vi "BioFeedback23(v_0.4).vi"() -> ()   [LabVIEW 2016]
doc: "Use this template to build a producer/consumer design pattern. Use this template when you need to execute a process, such as data analysis, when a data source, such as a triggered acquisition, produces data at an uneven rate and you need to execute the process when the data becomes available."
uses:
  customSubVIs/8ChanWfmArray.ctl
  <vilib>/Utility/file.llb/Write Delimited Spreadsheet (string).vi
panel:
  out "RecordStartTime":timestamp
  out "startRecording":bool
  out "numChannels":dbl=20.0 caption="Lower Cut-Off"
  in  "Number of Channels":dbl=2.0 min=1.0 max=8.0 step=1.0
  out "DispQueueSize":dbl
  out "Display Values":dbl(graph)
  in  "Display Width for Data Stream":dbl(slide)=1.0 caption="Chart Width in Seconds" scale=0.1..10.0
  in  "infiniteTrial":bool=TRUE caption="Infinite Trial"
  out "MVC State":enum16{"Nothing", "Saved MVC", "NoSave MVC"}(ring)
  in  "MVC Delay (s)":dbl=3.0
  out "trial last time":timestamp
  out "mvc last time":timestamp
  in  "Display Width for MVC (s)":dbl(slide)=1.0 caption="Chart Width in Seconds" scale=0.1..10.0
  in  "Display Width for Current Trial":dbl(slide)=1.0 caption="Chart Width in Seconds" scale=0.1..10.0
  out "Current Trial (Filtered)":waveform(dbl)(graph)
  out "Current MVC (Filtered)":waveform(dbl)(graph)
  in  "enableSave":bool=TRUE caption="No Save      Save"
  in  "barOrGraph":bool=TRUE caption="Graph (under construction)       Bar"
  in  "Trial comment":string
  out "Collecting Data":bool
  in  "Display Min":dbl
  in  "Display Max":dbl=100.0
  in  "log filepath":path
  in  "Trial Duration (s)":dbl=3.0
  out "Trial Number":dbl
  in  "Session Name":string="Default"
  out "loopTime":dbl=30.0 caption="Upper Cut-Off"
  in  "trial display data":path
  out "Disp Data":cluster{"queue out":refnum<queue>, dbl, dbl}[](array[cluster])
  in  "Target Percentage":dbl=10.0
  out "Current Activation":dbl
  out "DisplayBarActivation":dbl(slide) caption="Percent Activation" max=1.0 scale=0.0..100.0
  in  "EMG Channel To Display":dbl=1.0
  out "MVC Data":cluster{"queue out":refnum<queue>, dbl, dbl}[](array[cluster])
  out "Trial Name":string="Test"
  in  "Data Directory":path=path "C:/Users/Tinggroup/Desktop/EMG Biofeedback System/LabviewFiles/Data"
  in  "MVC Number":dbl=3.0
  in  "MVC Duration (s)":dbl=3.0
  in  "Frames Per Second":dbl=30.0 caption="Upper Cut-Off"
  in  "EMG Input Device\nProduct Type":string="USB-6009"
  out "raw data":waveform(dbl)[](graph)
  out "dispSize":dbl=20.0 caption="Lower Cut-Off"
  out "mvcSize":dbl=300.0 caption="Upper Cut-Off"
  in  "MVC Window Size (s)":dbl=0.5
  in  "Display Window Size (s)":dbl=0.5
  in  "MVC Raw Path":path
  in  "trial raw data":path
  in  "trial filtered data":path
  in  "MVC Filtered Path":path
  in  "Sample rate (Hz)":dbl=1000.0 caption="Upper Cut-Off"
  out "fps":dbl=20.0 caption="Lower Cut-Off"
  out "rate":dbl=300.0 caption="Upper Cut-Off"
  in  "Set Parameters":bool
  out "lower":dbl=20.0 caption="Lower Cut-Off"
  out "upper":dbl=300.0 caption="Upper Cut-Off"
  in  "Lower Cut-Off":dbl=20.0
  in  "Upper Cut-Off":dbl=500.0
  in  "Mark":bool
  in  "End Trial":bool
  in  "Get MVC":bool
  in  "StartTrial":bool
  out "State":T1(ring)
  out "FilteredAndRectified":waveform(dbl)[](graph) caption="FilteredAndRectified Data By Channel"
  in  "stop":bool
  # "Behind The Scenes"
  # "Timing"
  # "Add trial comment\nBEFORE beginning trial"
  # "Off         On"
  # "Display Settings"
  # "Filtering"
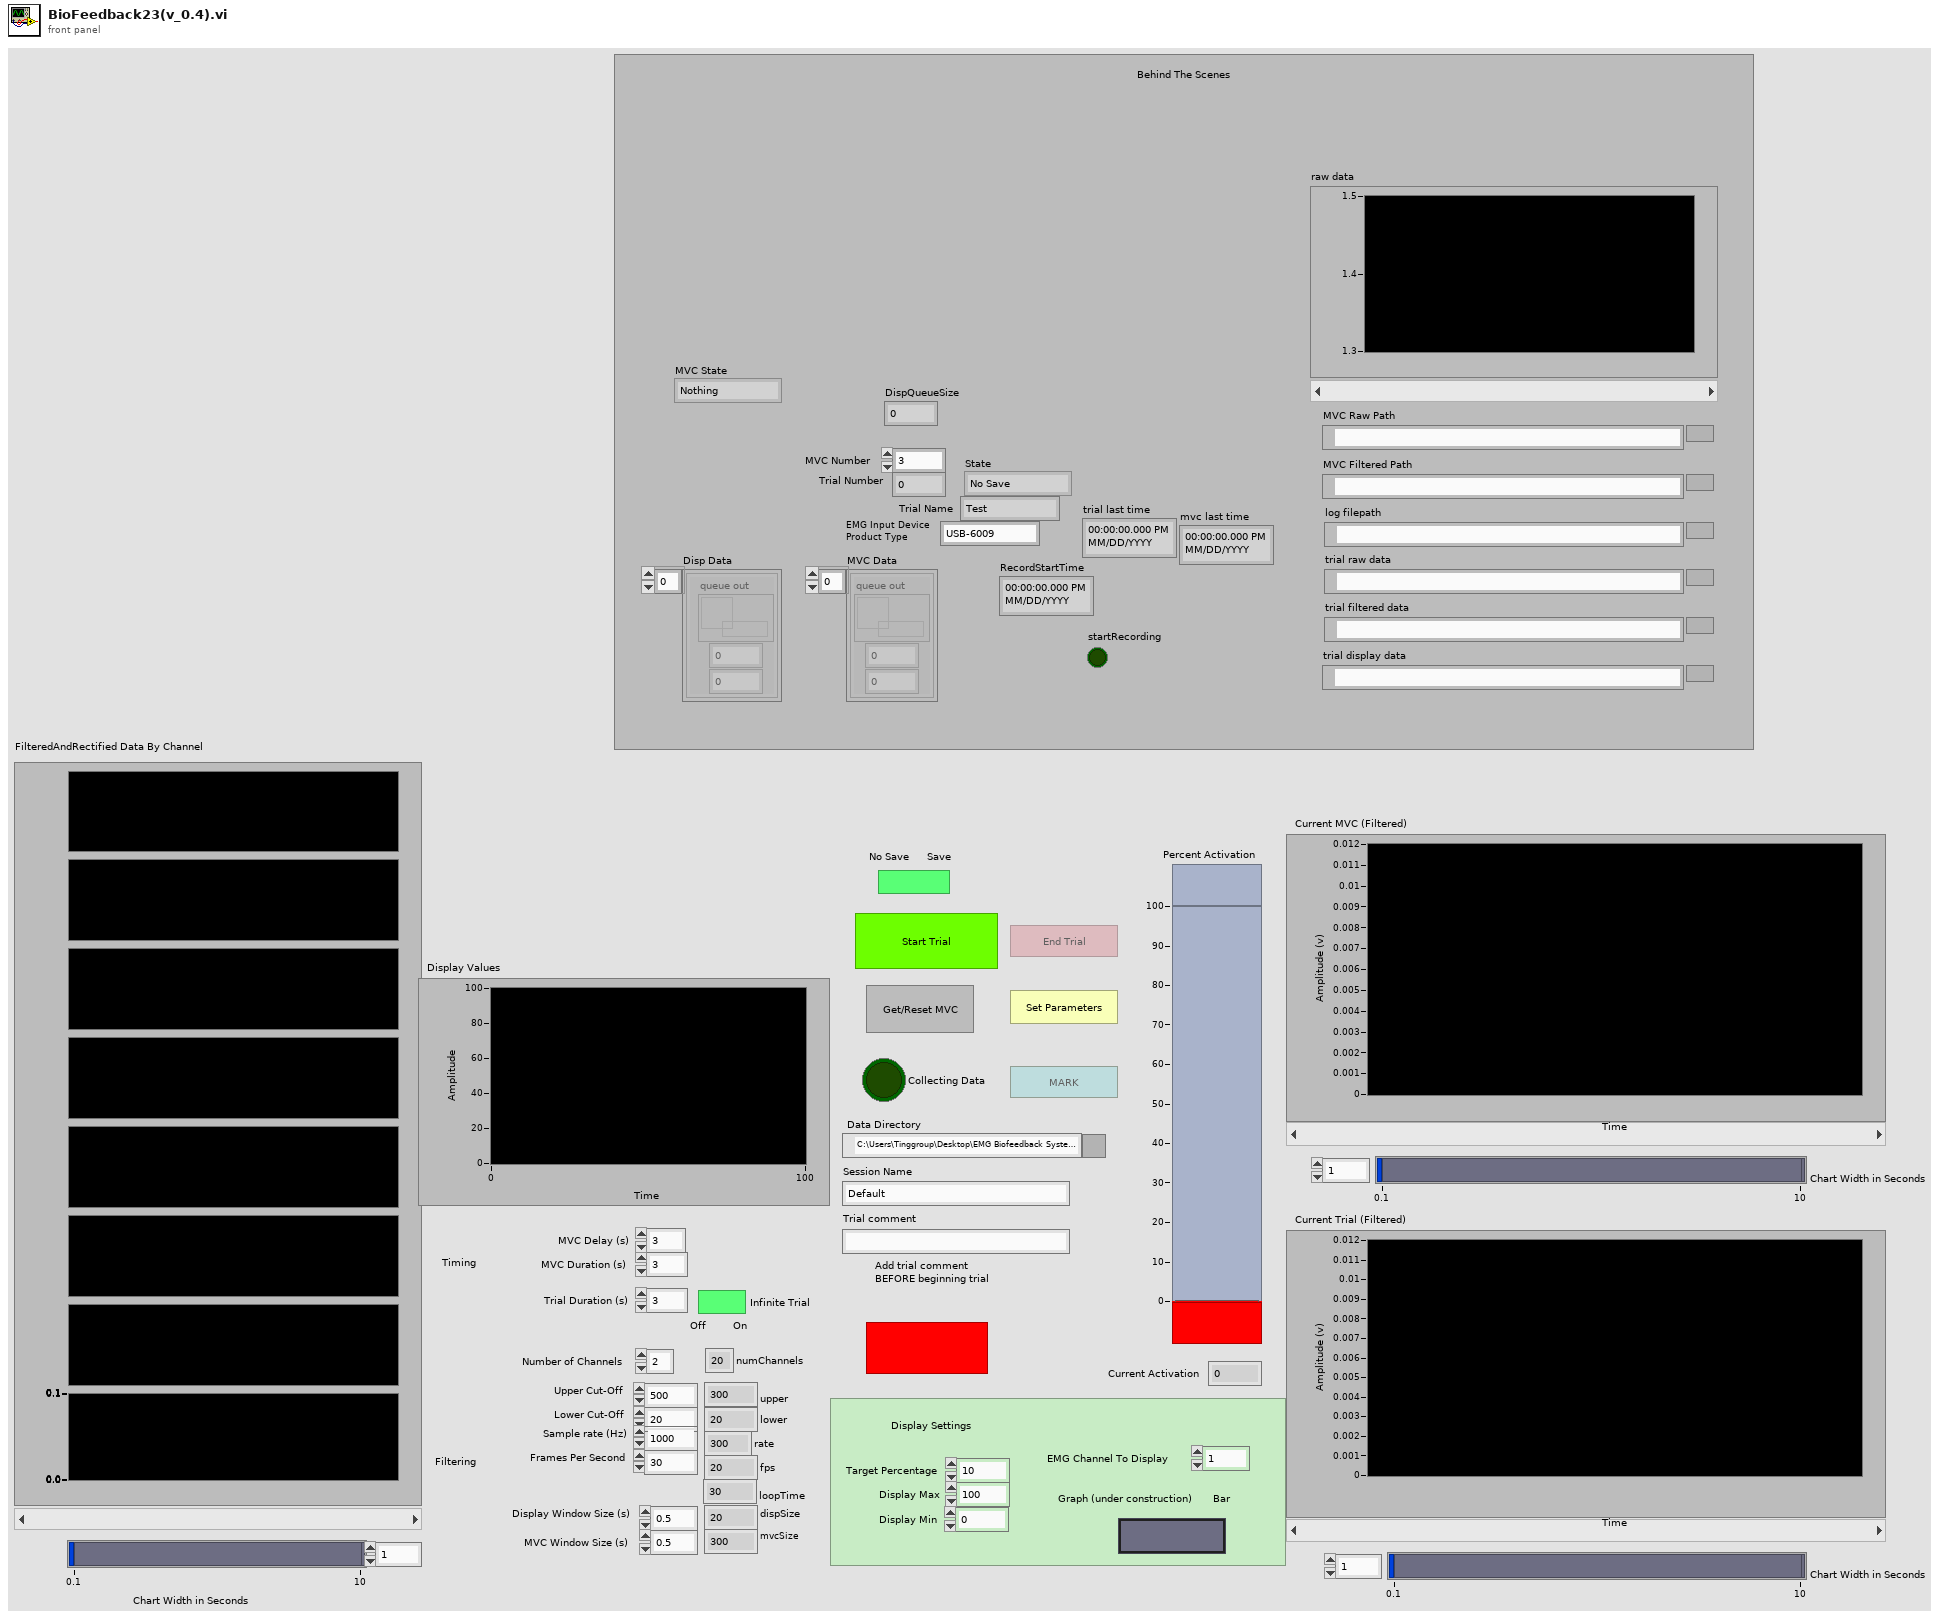
[diagram p1: front panel]
types:
  T1 = enum16{"No Save", "Acquiring Max", "Trial In Progress"}
  T2 = enum8{"Enabled", "Disabled", "Disabled and Grayed Out"}
  T3 = typedef "8ChanWfmArray.ctl" = waveform(dbl)[]
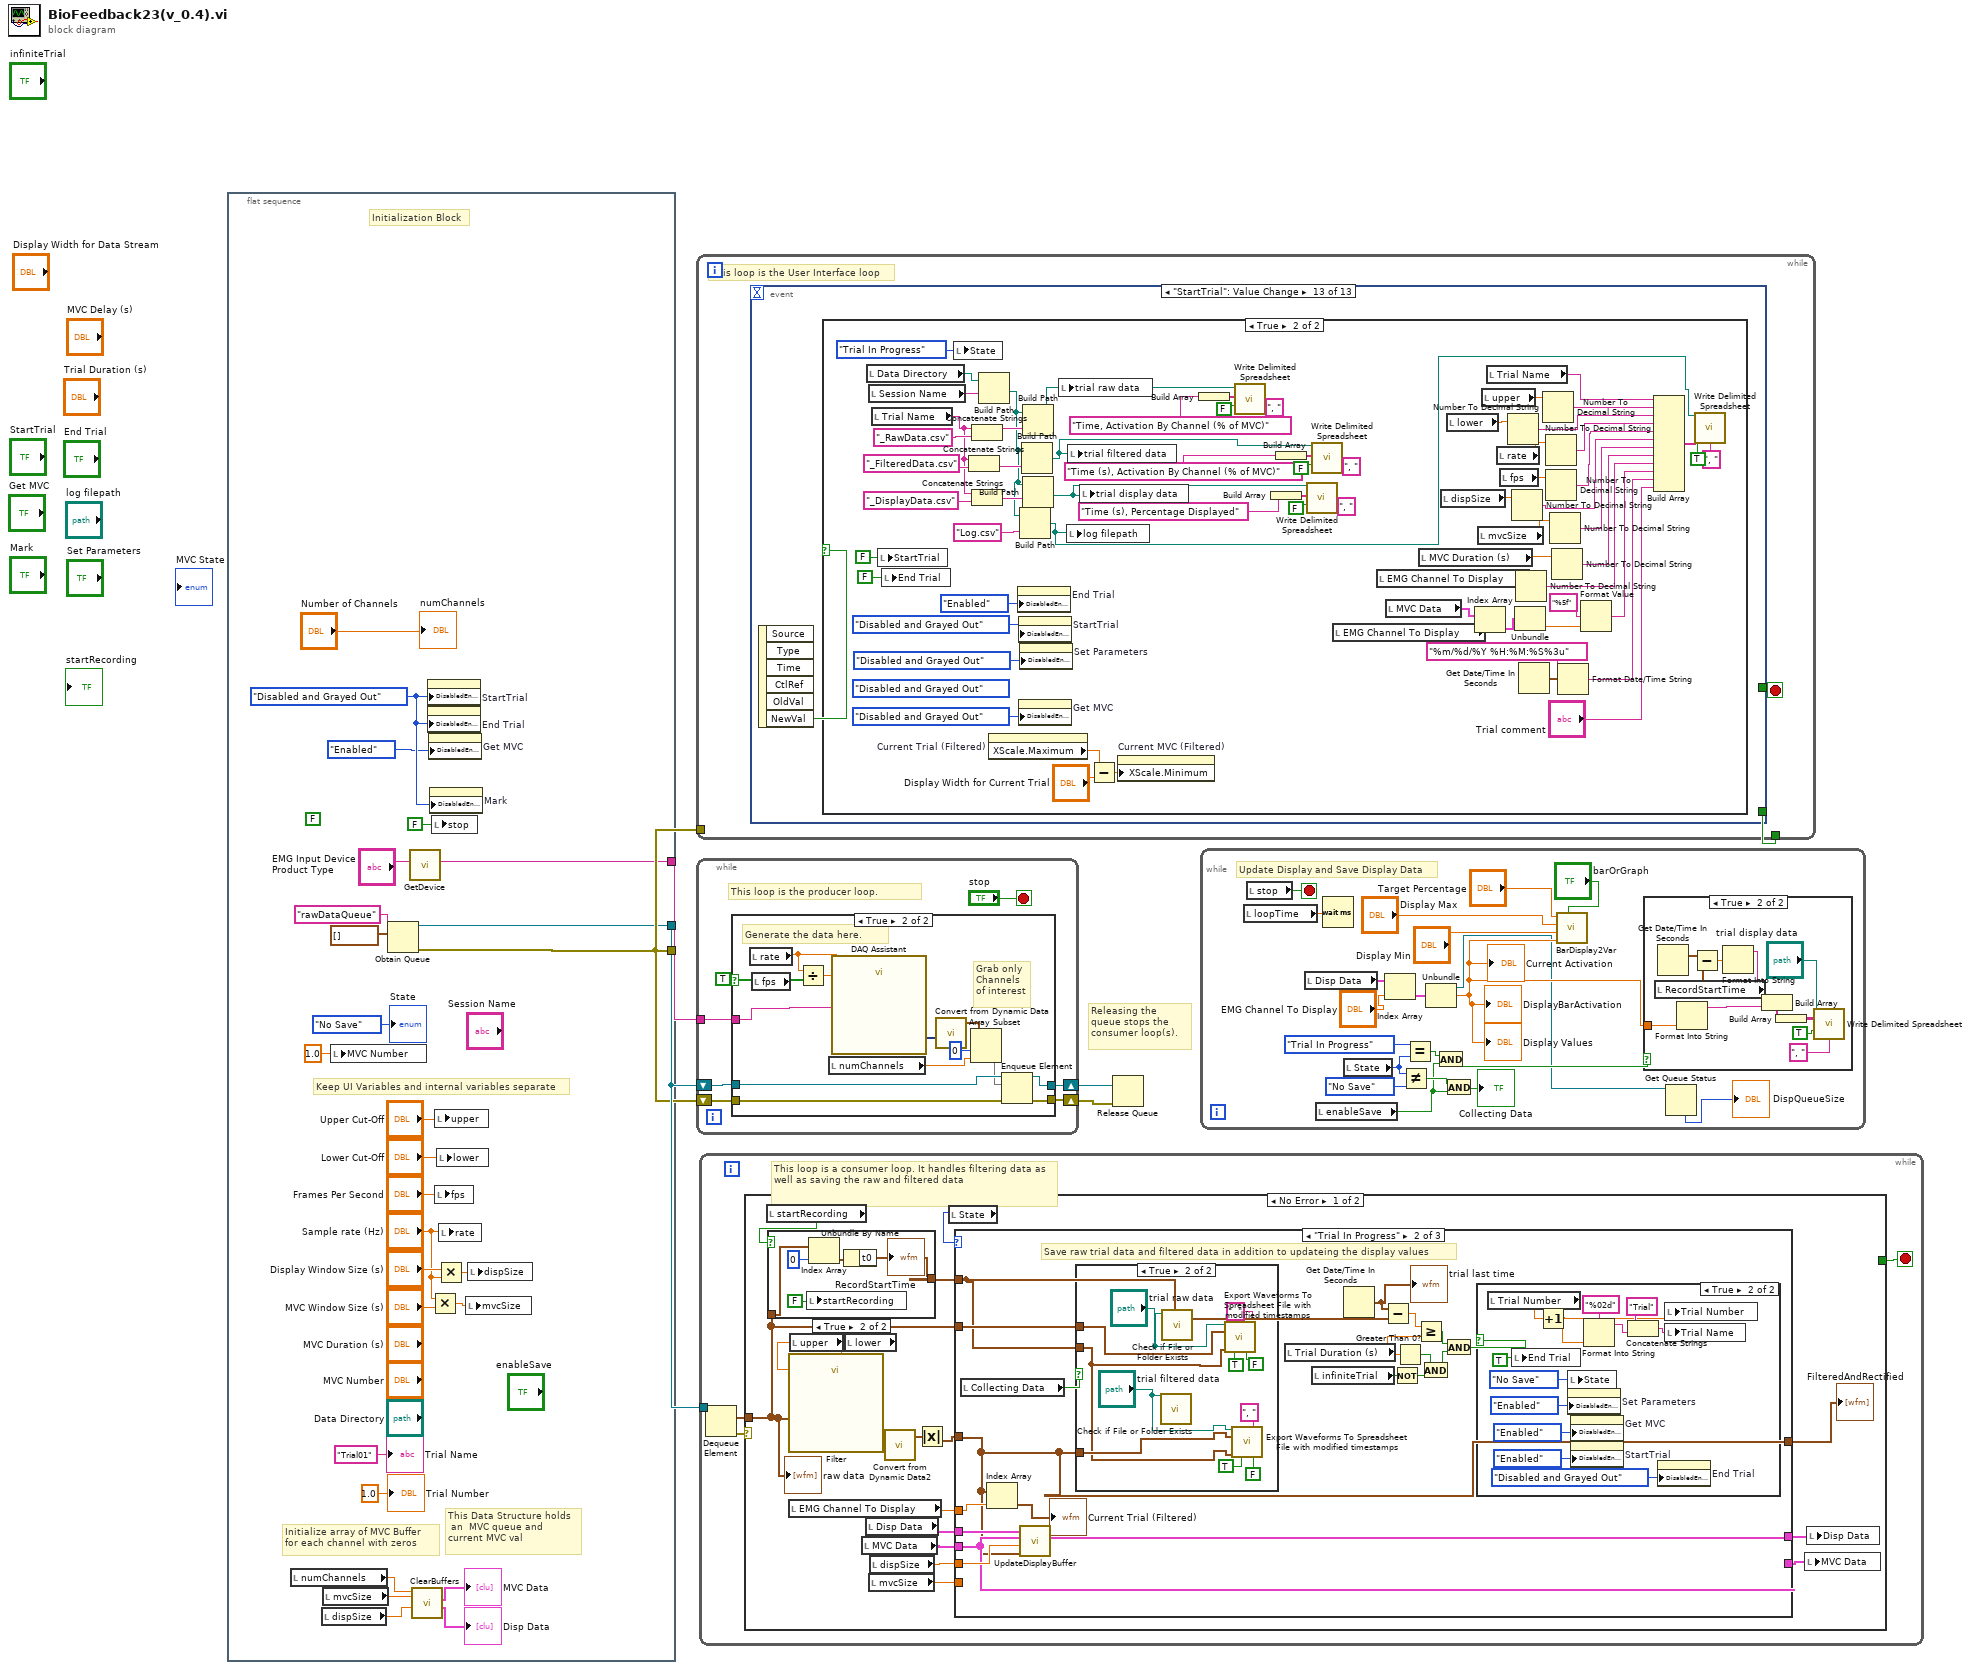
[diagram p0: block diagram]
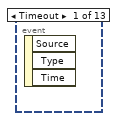
[diagram p3: hidden frame]
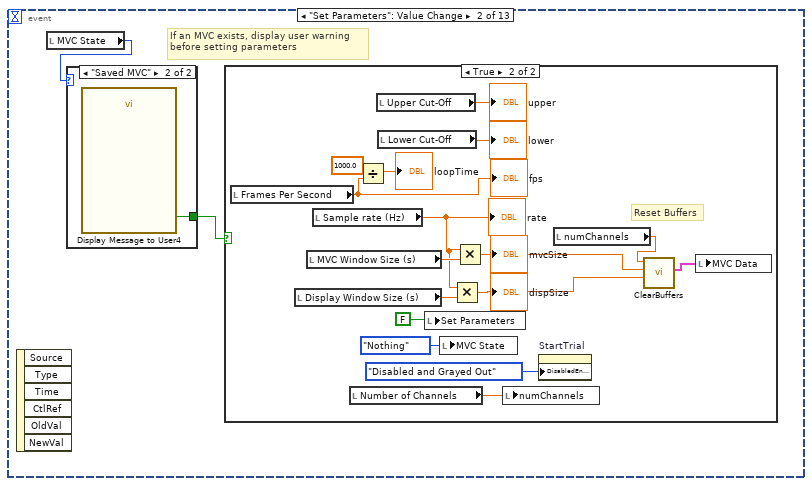
[diagram p4: hidden frame]
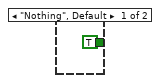
[diagram p6: hidden frame]
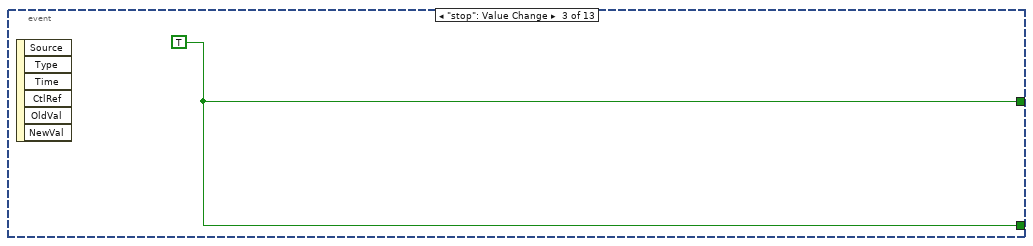
[diagram p7: hidden frame]
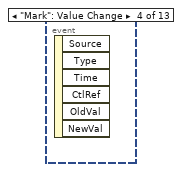
[diagram p8: hidden frame]
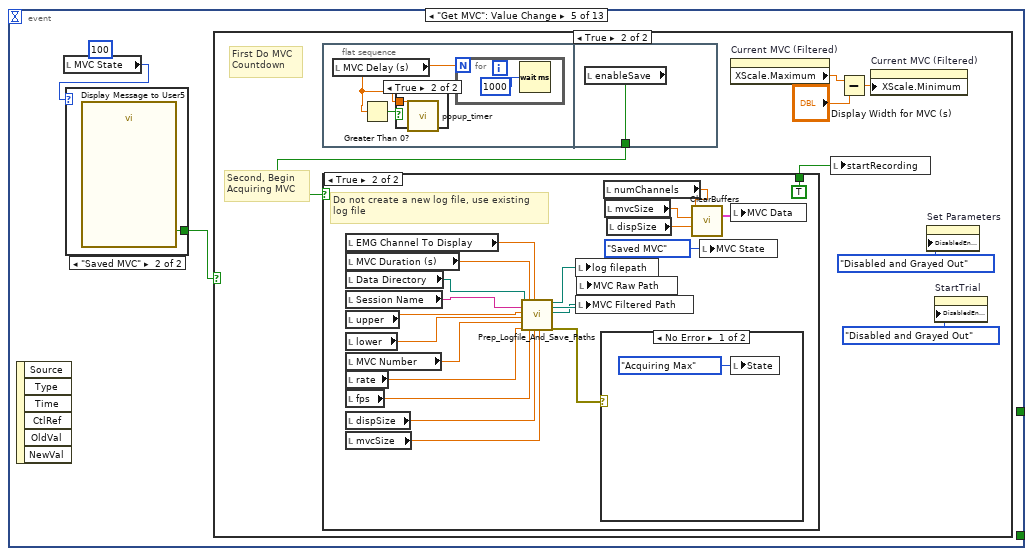
[diagram p9: hidden frame]
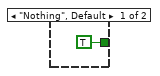
[diagram p10: hidden frame]
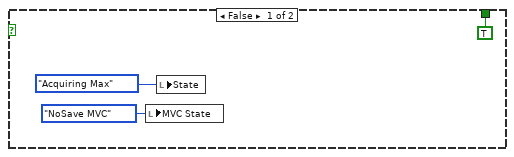
[diagram p13: hidden frame]
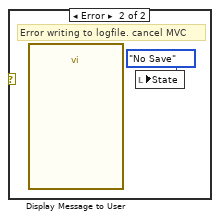
[diagram p14: hidden frame]
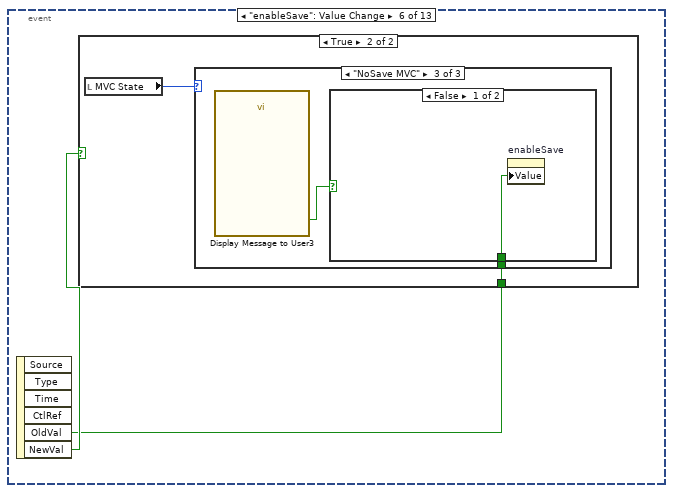
[diagram p15: hidden frame]
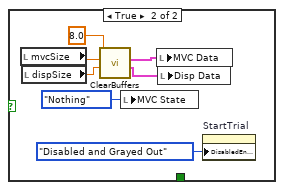
[diagram p19: hidden frame]
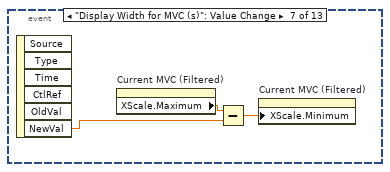
[diagram p20: hidden frame]
diagram:
  # "Releasing the\nqueue stops the consumer loop(s)."
  n1 = flat-sequence {
    tunnel: [w23] -> w2
    tunnel: [w22] -> w1
    tunnel: [w25] -> w3
    frame #0 {
      (unwired) FALSE ("Visible")
      w30 = T2."Disabled and Grayed Out" ("Disabled")
      # "Keep UI Variables and internal variables separate"
      # "This Data Structure holds\n an  MVC queue and \ncurrent MVC val"
      # "Initialize array of MVC Buffer \nfor each channel with zeros"
      # "Initialization Block"
      n2 = local read "numChannels"() -> (w6:dbl)
      n3 = local read "dispSize"() -> (w10:dbl)
      n4 = local read "mvcSize"() -> (w11:dbl)
      n5 = local write "MVC Number"(1.0 ("MVC Number")) -> ()
      n6 = Obtain Queue(name (unnamed)="rawDataQueue", element data type=T3 [] ("initialized array")) -> (queue out=w23:refnum<queue>, error out=w22:errorcluster)  [unwired: 3 in, 1 out]
      n7 = call "GetDevice.vi"("EMG Input Device\nProduct Type"="EMG Input Device\nProduct Type") -> ("DAQmx Device Name"=w25:tag)  [unwired: 10 in]
      n8 = call "ClearBuffers.vi"("disp size"=w10, "mvc size"=w11, "Num Channels"=w6) -> ("Disp Data"=→"Disp Data":cluster{"queue out":refnum<queue>, dbl, dbl}[], "MVC Data"=→"MVC Data":cluster{"queue out":refnum<queue>, dbl, dbl}[])  [unwired: 7 in]
      n9 = property on="StartTrial" class="Bool (strict)"("DisabledEnum"=w30) -> ()  [unwired: 2 in, 2 out]
      n10 = property on="End Trial" class="Bool (strict)"("DisabledEnum"=w30) -> ()  [unwired: 2 in, 2 out]
      n11 = property on="Get MVC" class="Bool"("DisabledEnum"=T2."Enabled" ("Disabled")) -> ()  [unwired: 2 in, 2 out]
      n12 = property on="Mark" class="Bool"("DisabledEnum"=w30) -> ()  [unwired: 2 in, 2 out]
      n13 = Multiply(x="Sample rate (Hz)", y="MVC Window Size (s)") -> (x*y=w17:dbl)
      n14 = local write "stop"(FALSE ("stop")) -> ()
      n15 = local write "upper"("Upper Cut-Off") -> ()
      n16 = local write "fps"("Frames Per Second") -> ()
      n17 = Multiply(x="Display Window Size (s)", y="Sample rate (Hz)") -> (x*y=w20:dbl)
      n18 = local write "lower"("Lower Cut-Off") -> ()
      n19 = local write "rate"("Sample rate (Hz)") -> ()
      n20 = local write "mvcSize"(w17) -> ()
      n21 = local write "dispSize"(w20) -> ()
      "Trial Name" <- "Trial01" ("Trial Name")
      "State" <- T1."No Save" ("State")
      "Trial Number" <- 1.0 ("Trial Number")
      "numChannels" <- "Number of Channels"
    }
  }
  n22 = while {
    tunnel: [w34] -> _
    tunnel: w1 -> [_]
    stop <- w33 stop-if-true
    # "This loop is the User Interface loop"
    n23 = event shown="[12] \"StartTrial\": Value Change" {
      selector: _ -> [_ _ _ _ _ _ _ _ _ _ _ _ _]
      dyn-events: _ -> [_ _ _ _ _ _ _ _ _ _ _ _ _]
      timeout: _ -> [_ _ _ _ _ _ _ _ _ _ _ _ _]
      tunnel: [_ _ w55 _ _ _ _ _ _ _ _ _ _] -> w33
      tunnel: [_ _ w55 _ _ _ _ _ _ _ _ _ _] -> w34
      event Timeout {
        n24 = event-data() -> ()  [unwired: 1 in, 3 out]
      }
      event "Set Parameters": Value Change {
        # "If an MVC exists, display user warning\nbefore setting parameters"
        n25 = event-data() -> ()  [unwired: 1 in, 6 out]
        n26 = local read "MVC State"() -> (w36:enum16{"Nothing", "Saved MVC", "NoSave MVC"})
        n27 = case shown="\"Saved MVC\"" w36 {
          tunnel: [TRUE ("Continue") w54] -> w35
          frame "Nothing", Default {
          }
          frame "Saved MVC" {
            n28 = call "Display Message to User4"() -> ("Continue"=w54:bool)  [unwired: 10 in, 1 out]
          }
        }
        n29 = case shown="True" w35 {
          frame False {
          }
          frame True {
            # "Reset Buffers"
            n30 = local read "Frames Per Second"() -> (w45:dbl)
            "fps" <- w45
            n31 = local read "Display Window Size (s)"() -> (w50:dbl)
            n32 = local read "MVC Window Size (s)"() -> (w51:dbl)
            n33 = local read "Sample rate (Hz)"() -> (w48:dbl)
            "rate" <- w48
            n34 = local read "Number of Channels"() -> (w37:dbl)
            n35 = Divide(x=1000.0, y=w45) -> (x/y=→"loopTime":dbl)
            n36 = local read "Upper Cut-Off"() -> (→"upper":dbl)
            n37 = local read "Lower Cut-Off"() -> (→"lower":dbl)
            n38 = local write "Set Parameters"(FALSE ("Set Parameters")) -> ()
            n39 = local write "MVC State"(enum16{"Nothing", "Saved MVC", "NoSave MVC"}."Nothing" ("MVC State")) -> ()
            n40 = Multiply(x=w48, y=w50) -> (x*y=w42:dbl)
            "dispSize" <- w42
            n41 = Multiply(x=w48, y=w51) -> (x*y=w43:dbl)
            "mvcSize" <- w43
            n42 = local write "numChannels"(w37) -> ()
            n43 = property on="StartTrial" class="Bool (strict)"("DisabledEnum"=T2."Disabled and Grayed Out" ("Disabled")) -> ()  [unwired: 2 in, 2 out]
            n44 = local read "numChannels"() -> (w38:dbl)
            n45 = call "ClearBuffers.vi"("disp size"=w42, "mvc size"=w43, "Num Channels"=w38) -> ("MVC Data"=w41:cluster{"queue out":refnum<queue>, dbl, dbl}[])  [unwired: 7 in, 1 out]
            n46 = local write "MVC Data"(w41) -> ()
          }
        }
      }
      event "stop": Value Change {
        w55 = TRUE
        n47 = event-data() -> ()  [unwired: 1 in, 6 out]
      }
      event "Mark": Value Change {
        n48 = event-data() -> ()  [unwired: 1 in, 6 out]
      }
      event "Get MVC": Value Change {
        (unwired) u32 100 ("milliseconds to wait")
        n49 = event-data() -> ()  [unwired: 1 in, 6 out]
        n50 = local read "MVC State"() -> (w57:enum16{"Nothing", "Saved MVC", "NoSave MVC"})
        n51 = case shown="\"Saved MVC\"" w57 {
          tunnel: [TRUE ("Continue") w59] -> w56
          frame "Nothing", Default {
          }
          frame "Saved MVC" {
            n52 = call "Display Message to User5"() -> ("Continue"=w59:bool)  [unwired: 10 in, 1 out]
          }
        }
        n53 = case shown="True" w56 {
          frame False {
          }
          frame True {
            # "Second, Begin \nAcquiring MVC"
            # "First Do MVC\nCountdown"
            n54 = flat-sequence {
              tunnel: [w71] -> w64
              frame #0 {
                n55 = local read "MVC Delay (s)"() -> (w67:dbl)
                n56 = Greater Than 0?(x=w67) -> (x > 0?=w68:bool)
                n57 = case shown="True" w68 {
                  tunnel: w67 -> [_ w69]
                  frame False {
                  }
                  frame True {
                    n58 = call "popup_timer.vi"("Seconds"=w69) -> ()  [unwired: 9 in, 1 out]
                  }
                }
                n59 = for {
                  N: w67 -> [_]
                  n60 = Wait (ms)(milliseconds to wait=u32 1000) -> ()  [unwired: 1 out]
                }
              }
              frame #1 {
                n61 = local read "enableSave"() -> (w71:bool)
              }
            }
            n62 = case shown="True" w64 {
              tunnel: [TRUE TRUE ("recordPressed")] -> w60
              frame False {
                n63 = local write "MVC State"(enum16{"Nothing", "Saved MVC", "NoSave MVC"}."NoSave MVC" ("MVC State")) -> ()
                n64 = local write "State"(T1."Acquiring Max" ("State")) -> ()
              }
              frame True {
                # "Do not create a new log file, use existing \nlog file"
                n65 = local read "EMG Channel To Display"() -> (w79:dbl)
                n66 = local read "MVC Duration (s)"() -> (w80:dbl)
                n67 = local read "Data Directory"() -> (w92:path)
                n68 = local read "Session Name"() -> (w91:string)
                n69 = local read "upper"() -> (w88:dbl)
                n70 = local read "lower"() -> (w87:dbl)
                n71 = local read "MVC Number"() -> (w86:dbl)
                n72 = local read "rate"() -> (w84:dbl)
                n73 = local read "fps"() -> (w83:dbl)
                n74 = local read "dispSize"() -> (w82:dbl)
                n75 = local read "mvcSize"() -> (w81:dbl)
                n76 = call "Prep_Logfile_And_Save_Paths.vi"("Data Directory"=w92, "Session Name"=w91, "upper"=w88, "lower"=w87, "MVC Number"=w86, "rate"=w84, "MVC Duration (s)"=w80, "fps"=w83, "EMG Channel To Display"=w79, "dispSize"=w82, "mvcSize"=w81) -> ("log filepath"=w90:path, "MVC Raw Path"=w89:path, "MVC Filtered Path"=w85:path, "error out"=w78:errorcluster)  [unwired: 4 in, 1 out]
                n77 = local write "log filepath"(w90) -> ()
                n78 = local write "MVC Filtered Path"(w85) -> ()
                n79 = local write "MVC Raw Path"(w89) -> ()
                n80 = case shown="No Error" w78 {
                  frame No Error {
                    n81 = local write "State"(T1."Acquiring Max" ("State")) -> ()
                  }
                  frame Error {
                    # "Error writing to logfile. cancel MVC"
                    n82 = call "Display Message to User"() -> ()  [unwired: 10 in, 2 out]
                    n83 = local write "State"(T1."No Save" ("State")) -> ()
                  }
                }
                n84 = local read "numChannels"() -> (w76:dbl)
                n85 = local read "mvcSize"() -> (w94:dbl)
                n86 = local read "dispSize"() -> (w93:dbl)
                n87 = call "ClearBuffers.vi"("disp size"=w93, "mvc size"=w94, "Num Channels"=w76) -> ("MVC Data"=w95:cluster{"queue out":refnum<queue>, dbl, dbl}[])  [unwired: 7 in, 1 out]
                n88 = local write "MVC State"(enum16{"Nothing", "Saved MVC", "NoSave MVC"}."Saved MVC" ("MVC State")) -> ()
                n89 = local write "MVC Data"(w95) -> ()
              }
            }
            n90 = property on="Current MVC (Filtered)" class="WFChart (strict)"() -> ("XScale.Maximum"=w61:dbl)  [unwired: 2 in, 2 out]
            n91 = local write "startRecording"(w60) -> ()
            n92 = Subtract(x=w61, y="Display Width for MVC (s)") -> (x-y=w63:dbl)
            n93 = property on="Current MVC (Filtered)" class="WFChart (strict)"("XScale.Minimum"=w63) -> ()  [unwired: 2 in, 2 out]
            n94 = property on="Set Parameters" class="Bool (strict)"("DisabledEnum"=T2."Disabled and Grayed Out" ("Disabled")) -> ()  [unwired: 2 in, 2 out]
            n95 = property on="StartTrial" class="Bool (strict)"("DisabledEnum"=T2."Disabled and Grayed Out" ("Disabled")) -> ()  [unwired: 2 in, 2 out]
          }
        }
      }
      event "enableSave": Value Change {
        n96 = event-data() -> ("OldVal"=w98:bool, "NewVal"=w99:bool)  [unwired: 1 in, 4 out]
        n97 = case shown="True" w99 {
          tunnel: w98 -> [_ w100]
          frame False {
          }
          frame True {
            n98 = local read "MVC State"() -> (w101:enum16{"Nothing", "Saved MVC", "NoSave MVC"})
            n99 = case shown="\"NoSave MVC\"" w101 {
              tunnel: w100 -> [_ _ w102]
              frame "Nothing", Default {
              }
              frame "Saved MVC" {
              }
              frame "NoSave MVC" {
                n100 = call "Display Message to User3"() -> ("Enable Saving"=w103:bool)  [unwired: 10 in, 1 out]
                n101 = case shown="False" w103 {
                  tunnel: w102 -> [w104 _]
                  frame False {
                    n102 = property on="enableSave" class="Bool (strict)"("Value"=w104) -> ()  [unwired: 2 in, 2 out]
                  }
                  frame True {
                    n103 = local read "mvcSize"() -> (w109:dbl)
                    n104 = local read "dispSize"() -> (w108:dbl)
                    n105 = call "ClearBuffers.vi"("disp size"=w108, "mvc size"=w109, "Num Channels"=8.0) -> ("Disp Data"=w111:cluster{"queue out":refnum<queue>, dbl, dbl}[], "MVC Data"=w110:cluster{"queue out":refnum<queue>, dbl, dbl}[])  [unwired: 7 in]
                    n106 = local write "MVC State"(enum16{"Nothing", "Saved MVC", "NoSave MVC"}."Nothing" ("MVC State")) -> ()
                    n107 = local write "MVC Data"(w110) -> ()
                    n108 = local write "Disp Data"(w111) -> ()
                    n109 = property on="StartTrial" class="Bool (strict)"("DisabledEnum"=T2."Disabled and Grayed Out" ("Disabled")) -> ()  [unwired: 2 in, 2 out]
                  }
                }
              }
            }
          }
        }
      }
      event "Display Width for MVC (s)": Value Change {
        n110 = event-data() -> ("NewVal"=w114:dbl)  [unwired: 1 in, 5 out]
        n111 = property on="Current MVC (Filtered)" class="WFChart (strict)"() -> ("XScale.Maximum"=w112:dbl)  [unwired: 2 in, 2 out]
        n112 = Subtract(x=w112, y=w114) -> (x-y=w113:dbl)
        n113 = property on="Current MVC (Filtered)" class="WFChart (strict)"("XScale.Minimum"=w113) -> ()  [unwired: 2 in, 2 out]
      }
      event "Display Width for Current Trial": Value Change {
        n114 = event-data() -> ("NewVal"=w117:dbl)  [unwired: 1 in, 5 out]
        n115 = property on="Current Trial (Filtered)" class="WFChart (strict)"() -> ("XScale.Maximum"=w115:dbl)  [unwired: 2 in, 2 out]
        n116 = Subtract(x=w115, y=w117) -> (x-y=w116:dbl)
        n117 = property on="Current Trial (Filtered)" class="WFChart (strict)"("XScale.Minimum"=w116) -> ()  [unwired: 2 in, 2 out]
      }
      event "Display Width for Data Stream": Value Change {
        n118 = event-data() -> ("NewVal"=w118:dbl)  [unwired: 1 in, 5 out]
        n119 = property on="raw data" class="WFChart (strict)"() -> ("XScale.Maximum"=w119:dbl)  [unwired: 2 in, 2 out]
        n120 = property on="FilteredAndRectified" class="WFChart (strict)"() -> ("XScale.Maximum"=w121:dbl)  [unwired: 2 in, 2 out]
        n121 = Subtract(x=w121, y=w118) -> (x-y=w120:dbl)
        n122 = Subtract(x=w119, y=w118) -> (x-y=w122:dbl)
        n123 = property on="raw data" class="WFChart (strict)"("XScale.Minimum"=w122) -> ()  [unwired: 2 in, 2 out]
        n124 = property on="FilteredAndRectified" class="WFChart (strict)"("XScale.Minimum"=w120) -> ()  [unwired: 2 in, 2 out]
      }
      event "infiniteTrial": Value Change {
        n125 = event-data() -> ("NewVal"=w123:bool)  [unwired: 1 in, 5 out]
        n126 = case shown="False" w123 {
          tunnel: [T2."Enabled" ("Disabled") T2."Disabled and Grayed Out" ("Disabled")] -> w124
          frame False {
          }
          frame True {
          }
        }
        n127 = property on="Trial Duration (s)" class="DigNum (strict)"("DisabledEnum"=w124) -> ()  [unwired: 2 in, 2 out]
      }
      event "Session Name": Value Change {
        # "Only Prompot if MVC already exists"
        # "Dialog Prompt User if they are sure that they want to change sessionname"
        n128 = event-data() -> ("OldVal"=w128:string)  [unwired: 1 in, 5 out]
        n129 = local read "MVC State"() -> (w127:enum16{"Nothing", "Saved MVC", "NoSave MVC"})
        n130 = case shown="\"Saved MVC\"" w127 {
          tunnel: w128 -> [_ w129]
          frame "Nothing", Default {
          }
          frame "Saved MVC" {
            n131 = call "Display Message to User2"() -> ("Change"=w130:bool)  [unwired: 10 in, 1 out]
            n132 = case shown="True" w130 {
              tunnel: w129 -> [w132 _]
              frame False {
                # "User cancels"
                n133 = Variant To Data(Variant=w132) -> (data=w131:string)  [unwired: 2 in, 1 out]
                n134 = local write "Session Name"(w131) -> ()
              }
              frame True {
                # "User Continues. Reset MVC"
                n135 = local read "numChannels"() -> (w133:dbl)
                n136 = local read "mvcSize"() -> (w138:dbl)
                n137 = local read "dispSize"() -> (w137:dbl)
                n138 = call "ClearBuffers.vi"("disp size"=w137, "mvc size"=w138, "Num Channels"=w133) -> ("Disp Data"=w135:cluster{"queue out":refnum<queue>, dbl, dbl}[], "MVC Data"=w136:cluster{"queue out":refnum<queue>, dbl, dbl}[])  [unwired: 7 in]
                n139 = local write "MVC State"(enum16{"Nothing", "Saved MVC", "NoSave MVC"}."Nothing" ("MVC State")) -> ()
                n140 = local write "MVC Data"(w136) -> ()
                n141 = local write "Disp Data"(w135) -> ()
                n142 = property on="StartTrial" class="Bool (strict)"("DisabledEnum"=T2."Disabled and Grayed Out" ("Disabled")) -> ()  [unwired: 2 in, 2 out]
              }
            }
          }
        }
      }
      event "End Trial": Value Change {
        n143 = event-data() -> ("NewVal"=w140:bool)  [unwired: 1 in, 5 out]
        n144 = case shown="True" w140 {
          frame False {
          }
          frame True {
            (unwired) T2."Enabled" ("Disabled")
            n145 = local read "Trial Number"() -> (w145:dbl)
            n146 = Increment(x=w145) -> (x+1=w141:dbl)
            n147 = local write "State"(T1."No Save" ("State")) -> ()
            n148 = Format Into String(format string="%02d", w141) -> (resulting string=w144:string)  [unwired: 2 in, 1 out]
            n149 = local write "Trial Number"(w141) -> ()
            n150 = Concatenate Strings("Trial" ("string"), w144) -> (w146:string)
            n151 = property on="End Trial" class="Bool (strict)"("DisabledEnum"=T2."Disabled and Grayed Out" ("Disabled")) -> ()  [unwired: 2 in, 2 out]
            n152 = property on="Get MVC" class="Bool"("DisabledEnum"=T2."Enabled" ("Disabled")) -> ()  [unwired: 2 in, 2 out]
            n153 = property on="Set Parameters" class="Bool (strict)"("DisabledEnum"=T2."Enabled" ("Disabled")) -> ()  [unwired: 2 in, 2 out]
            n154 = property on="StartTrial" class="Bool (strict)"("DisabledEnum"=T2."Enabled" ("Disabled")) -> ()  [unwired: 2 in, 2 out]
            n155 = local write "End Trial"(FALSE ("End Trial")) -> ()
            n156 = local write "Trial Name"(w146) -> ()
          }
        }
      }
      event "StartTrial": Value Change {
        n157 = event-data() -> ("NewVal"=w153:bool)  [unwired: 1 in, 5 out]
        n158 = case shown="True" w153 {
          frame False {
          }
          frame True {
            (unwired) T2."Disabled and Grayed Out" ("Disabled")
            n159 = local read "Data Directory"() -> (w213:path)
            n160 = local read "Session Name"() -> (w212:string)
            n161 = local read "Trial Name"() -> (w199:string)
            n162 = local write "StartTrial"(FALSE ("StartTrial")) -> ()
            n163 = local write "End Trial"(FALSE ("End Trial")) -> ()
            n164 = local write "State"(T1."Trial In Progress" ("State")) -> ()
            n165 = Concatenate Strings(w199, "_FilteredData.csv" ("string")) -> (w217:string)
            n166 = Concatenate Strings(w199, "_RawData.csv" ("string")) -> (w215:string)
            n167 = Concatenate Strings(w199, "_DisplayData.csv" ("string")) -> (w219:string)
            n168 = Build Path(base path=w213, name or relative path=w212) -> (appended path=w198:path)
            n169 = property on="Current Trial (Filtered)" class="WFChart (strict)"() -> ("XScale.Maximum"=w169:dbl)  [unwired: 2 in, 2 out]
            n170 = property on="End Trial" class="Bool (strict)"("DisabledEnum"=T2."Enabled" ("Disabled")) -> ()  [unwired: 2 in, 2 out]
            n171 = property on="StartTrial" class="Bool (strict)"("DisabledEnum"=T2."Disabled and Grayed Out" ("Disabled")) -> ()  [unwired: 2 in, 2 out]
            n172 = property on="Get MVC" class="Bool"("DisabledEnum"=T2."Disabled and Grayed Out" ("Disabled")) -> ()  [unwired: 2 in, 2 out]
            n173 = Build Path(base path=w198, name or relative path="Log.csv" ("string")) -> (appended path=w182:path)
            n174 = property on="Set Parameters" class="Bool (strict)"("DisabledEnum"=T2."Disabled and Grayed Out" ("Disabled")) -> ()  [unwired: 2 in, 2 out]
            n175 = Build Path(base path=w198, name or relative path=w217) -> (appended path=w160:path)
            n176 = Build Path(base path=w198, name or relative path=w215) -> (appended path=w164:path)
            n177 = Build Path(base path=w198, name or relative path=w219) -> (appended path=w155:path)
            n178 = local write "trial raw data"(w164) -> ()
            n179 = local write "log filepath"(w182) -> ()
            n180 = local write "trial filtered data"(w160) -> ()
            n181 = local write "trial display data"(w155) -> ()
            n182 = Subtract(x=w169, y="Display Width for Current Trial") -> (x-y=w171:dbl)
            n183 = property on="Current MVC (Filtered)" class="WFChart (strict)"("XScale.Minimum"=w171) -> ()  [unwired: 2 in, 2 out]
            n184 = Build Array("Time, Activation By Channel (% of MVC)" ("time format string (%c)")) -> (w166:string[])
            n185 = call-poly <vilib>:"Write Delimited Spreadsheet.vi"("file path (dialog if empty)"=w164, "1D data"=w166, "append to file? (new file:F)"=FALSE, "delimiter (\\t)"=", " ("delimiter (\\t)")) -> ()  [unwired: 10 in, 2 out]
            n186 = Build Array("Time (s), Percentage Displayed" ("time format string (%c)")) -> (w156:string[])
            n187 = Build Array("Time (s), Activation By Channel (% of MVC)" ("time format string (%c)")) -> (w161:string[])
            n188 = call-poly <vilib>:"Write Delimited Spreadsheet.vi"("file path (dialog if empty)"=w155, "1D data"=w156, "append to file? (new file:F)"=FALSE, "delimiter (\\t)"=", " ("delimiter (\\t)")) -> ()  [unwired: 10 in, 2 out]
            n189 = call-poly <vilib>:"Write Delimited Spreadsheet.vi"("file path (dialog if empty)"=w160, "1D data"=w161, "append to file? (new file:F)"=FALSE, "delimiter (\\t)"=", " ("delimiter (\\t)")) -> ()  [unwired: 10 in, 2 out]
            n190 = local read "EMG Channel To Display"() -> (w178:dbl)
            n191 = local read "EMG Channel To Display"() -> (w208:dbl)
            n192 = local read "MVC Data"() -> (w179:cluster{"queue out":refnum<queue>, dbl, dbl}[])
            n193 = local read "MVC Duration (s)"() -> (w207:dbl)
            n194 = local read "dispSize"() -> (w205:dbl)
            n195 = local read "lower"() -> (w202:dbl)
            n196 = Index Array(array=w179, index=w178) -> (element=w177:cluster{"queue out":refnum<queue>, dbl, dbl})
            n197 = local read "mvcSize"() -> (w206:dbl)
            n198 = local read "upper"() -> (w201:dbl)
            n199 = local read "Trial Name"() -> (w195:string)
            n200 = local read "rate"() -> (w203:dbl)
            n201 = local read "fps"() -> (w204:dbl)
            n202 = Number To Decimal String(number=w202) -> (decimal integer string=w191:string)  [unwired: 1 in]
            n203 = Number To Decimal String(number=w205) -> (decimal integer string=w189:string)  [unwired: 1 in]
            n204 = Unbundle(w177) -> (w173:dbl)  [unwired: 2 out]
            n205 = Number To Decimal String(number=w208) -> (decimal integer string=w186:string)  [unwired: 1 in]
            n206 = Get Date/Time In Seconds() -> (seconds since 1Jan1904=w181:timestamp)
            n207 = Number To Decimal String(number=w201) -> (decimal integer string=w192:string)  [unwired: 1 in]
            n208 = Number To Decimal String(number=w203) -> (decimal integer string=w190:string)  [unwired: 1 in]
            n209 = Number To Decimal String(number=w204) -> (decimal integer string=w185:string)  [unwired: 1 in]
            n210 = Number To Decimal String(number=w206) -> (decimal integer string=w188:string)  [unwired: 1 in]
            n211 = Number To Decimal String(number=w207) -> (decimal integer string=w187:string)  [unwired: 1 in]
            n212 = Format Date/Time String(time format string (%c)="%m/%d/%Y %H:%M:%S%3u", seconds (now)=w181) -> (date/time string=w176:string)  [unwired: 1 in]
            n213 = Format Value(format string="%5f", value (0)=w173) -> (output string=w172:string)  [unwired: 1 in]
            n214 = Build Array(w195, w192, w191, w190, w185, w189, w188, w187, w186, w172, w176, "Trial comment") -> (w184:string[])
            n215 = call-poly <vilib>:"Write Delimited Spreadsheet.vi"("file path (dialog if empty)"=w182, "1D data"=w184, "append to file? (new file:F)"=TRUE, "delimiter (\\t)"=", " ("delimiter (\\t)")) -> ()  [unwired: 10 in, 2 out]
          }
        }
      }
    }
  }
  n216 = while {
    shift-right: [w224] -> w4
    shift-left: w1 -> [w225]
    shift-right: [w221] -> w5
    shift-left: w2 -> [w226]
    tunnel: w3 -> [w222]
    stop <- "stop" stop-if-true
    # "This loop is the producer loop."
    n217 = case shown="True" TRUE ("Case Constant\n(See Context Help)") {
      tunnel: w226 -> [w228 w237]
      tunnel: w225 -> [w229 w242]
      tunnel: [w229 w241] -> w224
      tunnel: w222 -> [_ w234]
      tunnel: [w228 w236] -> w221
      frame False {
      }
      frame True {
        # "Grab only\nChannels \nof interest"
        # "Generate the data here."
        n218 = local read "rate"() -> (w239:dbl)
        n219 = local read "fps"() -> (w240:dbl)
        n220 = Divide(x=w239, y=w240) -> (x/y=w238:dbl)
        n221 = local read "numChannels"() -> (w232:dbl)
        n222 = call "DAQ Assistant"("rate"=w239, "number of samples"=w238, "device name"=w234) -> ("data"=w233:dynamicdata)  [unwired: 13 in, 3 out]
        n223 = call "Convert from Dynamic Data"("Dynamic Data Type"=w233) -> ("Array of Waveform"=w231:waveform(dbl)[])  [unwired: 3 in]
        n224 = Array Subset(array=w231, index=0, length=w232) -> (w230:waveform(dbl)[])
        n225 = Enqueue Element(queue=w237, element=w230, error in (no error)=w242) -> (queue out=w236:refnum<queue>, error out=w241:errorcluster)  [unwired: 1 in, 1 out]
      }
    }
  }
  n226 = while {
    tunnel: w2 -> [w243]
    stop <- w244 stop-if-true
    # "This loop is a consumer loop. It handles filtering data as well as saving the raw and filtered data"
    n227 = Dequeue Element(queue=w243) -> (element=w245:T3, error out=w246:errorcluster)  [unwired: 2 in, 2 out]
    n228 = case shown="No Error" w246 {
      tunnel: w245 -> [w247 _]
      tunnel: [_ TRUE] -> w244
      frame No Error {
        n229 = local read "startRecording"() -> (w249:bool)
        n230 = case shown="True" w249 {
          tunnel: [w264 w268] -> w248
          tunnel: w247 -> [_ w267]
          frame False {
            n231 = local read "RecordStartTime"() -> (w264:timestamp)
          }
          frame True {
            n232 = local write "startRecording"(FALSE) -> ()
            n233 = Index Array(array=w267, index=0) -> (element=w265:waveform(dbl))
            n234 = Unbundle By Name(w265) -> ("t0"=w268:timestamp)
            "RecordStartTime" <- w268
          }
        }
        n235 = local read "EMG Channel To Display"() -> (w253:dbl)
        n236 = local read "upper"() -> (w261:dbl)
        n237 = local read "lower"() -> (w260:dbl)
        n238 = call "Filter"("Lower Cut-Off"=w260, "Upper Cut-Off"=w261, "Signal"=w247) -> ("Filtered Signal"=w262:dynamicdata)  [unwired: 7 in, 1 out]
        n239 = local read "MVC Data"() -> (w258:cluster{"queue out":refnum<queue>, dbl, dbl}[])
        n240 = local read "Disp Data"() -> (w257:cluster{"queue out":refnum<queue>, dbl, dbl}[])
        n241 = local read "mvcSize"() -> (w251:dbl)
        n242 = local read "dispSize"() -> (w252:dbl)
        n243 = call "Convert from Dynamic Data2"("Dynamic Data Type"=w262) -> ("Array of Waveform"=w263:waveform(dbl)[])  [unwired: 3 in]
        n244 = Absolute Value(x=w263) -> (abs(x)=w259:waveform(dbl)[])
        n245 = local read "State"() -> (w254:T1)
        n246 = case shown="\"Trial In Progress\"" w254 {
          tunnel: w259 -> [w270 w276 w318]
          tunnel: w247 -> [_ w289 w329]
          tunnel: w258 -> [w273 w281 w324]
          tunnel: w257 -> [w274 w284 w325]
          tunnel: [w271 w282 w321] -> w255
          tunnel: [w273 w281 w320] -> w256
          tunnel: w253 -> [_ w287 w328]
          tunnel: w252 -> [w272 w283 w323]
          tunnel: w251 -> [_ _ w322]
          tunnel: [w270 w276 w318] -> w250
          tunnel: w248 -> [_ w275 w317]
          frame "No Save", Default {
            # "Update the display values, but do not save anything\n\nNote: MVC data is just referenced to calculate percent activation"
            n247 = call "UpdateDisplayBuffer.vi"("FilteredAndRectified"=w270, "dispSize"=w272, "MVC Data"=w273, "Disp Data"=w274) -> ("Disp Data Out"=w271:cluster{"queue out":refnum<queue>, dbl, dbl}[])  [unwired: 7 in]
          }
          frame "Trial In Progress" {
            # "Save raw trial data and filtered data in addition to updateing the display values"
            n248 = local read "Collecting Data"() -> (w288:bool)
            n249 = Index Array(array=w276, index=w287) -> (element=→"Current Trial (Filtered)":waveform(dbl))
            n250 = call "UpdateDisplayBuffer.vi"("FilteredAndRectified"=w276, "dispSize"=w283, "MVC Data"=w281, "Disp Data"=w284) -> ("Disp Data Out"=w282:cluster{"queue out":refnum<queue>, dbl, dbl}[])  [unwired: 7 in]
            n251 = case shown="True" w288 {
              tunnel: w276 -> [_ w302]
              tunnel: w289 -> [_ w296]
              tunnel: w275 -> [_ w297]
              frame False {
              }
              frame True {
                n252 = call <vilib>:"Check if File or Folder Exists.vi"("path"="trial filtered data") -> ()  [unwired: 8 in, 3 out]
                n253 = call <vilib>:"Check if File or Folder Exists.vi"("path"="trial raw data") -> ()  [unwired: 8 in, 3 out]
                n254 = call "Export Waveforms To Spreadsheet File with modified timestamps.vi"("file path (dialog if empty)"="trial raw data", "delimiter (Tab)"=", ", "waveforms"=w296, "trial start time"=w297, "append to file? (new file:F)"=TRUE, "header? (write header:T)"=FALSE) -> ()  [unwired: 8 in, 2 out]
                n255 = call "Export Waveforms To Spreadsheet File with modified timestamps.vi"("file path (dialog if empty)"="trial filtered data", "delimiter (Tab)"=", ", "waveforms"=w302, "trial start time"=w297, "append to file? (new file:F)"=TRUE, "header? (write header:T)"=FALSE) -> ()  [unwired: 8 in, 2 out]
              }
            }
            n256 = local read "Trial Duration (s)"() -> (w291:dbl)
            n257 = local read "infiniteTrial"() -> (w277:bool)
            n258 = Get Date/Time In Seconds() -> (seconds since 1Jan1904=w285:timestamp)
            "trial last time" <- w285
            n259 = Subtract(x=w285, y=w275) -> (x-y=w293:dbl)
            n260 = Not(x=w277) -> (.not. x?=w280:bool)
            n261 = Greater Than 0?(x=w291) -> (x > 0?=w279:bool)
            n262 = Greater Or Equal?(x=w293, y=w291) -> (x >= y?=w290:bool)
            n263 = And(x=w279, y=w280) -> (x .and. y?=w278:bool)
            n264 = And(x=w290, y=w278) -> (x .and. y?=w292:bool)
            n265 = case shown="True" w292 {
              frame False {
              }
              frame True {
                n266 = local read "Trial Number"() -> (w306:dbl)
                n267 = local write "End Trial"(TRUE ("End Trial")) -> ()
                n268 = Increment(x=w306) -> (x+1=w305:dbl)
                n269 = local write "State"(T1."No Save" ("State")) -> ()
                n270 = property on="Set Parameters" class="Bool (strict)"("DisabledEnum"=T2."Enabled" ("Disabled")) -> ()  [unwired: 2 in, 2 out]
                n271 = property on="Get MVC" class="Bool"("DisabledEnum"=T2."Enabled" ("Disabled")) -> ()  [unwired: 2 in, 2 out]
                n272 = property on="StartTrial" class="Bool (strict)"("DisabledEnum"=T2."Enabled" ("Disabled")) -> ()  [unwired: 2 in, 2 out]
                n273 = Format Into String(format string="%02d", w305) -> (resulting string=w311:string)  [unwired: 2 in, 1 out]
                n274 = Concatenate Strings("Trial" ("string"), w311) -> (w315:string)
                n275 = property on="End Trial" class="Bool (strict)"("DisabledEnum"=T2."Disabled and Grayed Out" ("Disabled")) -> ()  [unwired: 2 in, 2 out]
                n276 = local write "Trial Number"(w305) -> ()
                n277 = local write "Trial Name"(w315) -> ()
              }
            }
          }
          frame "Acquiring Max" {
            # "Automatically Stop Listening for Max\n after Acquire Max Time is elapsed"
            n278 = local read "Collecting Data"() -> (w330:bool)
            n279 = call "UpdateMovingAverages.vi"("FilteredAndRectified"=w318, "mvcSize"=w322, "dispSize"=w323, "MVC Data"=w324, "Disp Data"=w325) -> ("MVC Data Out"=w320:cluster{"queue out":refnum<queue>, dbl, dbl}[], "Disp Data Out"=w321:cluster{"queue out":refnum<queue>, dbl, dbl}[])  [unwired: 5 in]
            n280 = case shown="True" w330 {
              tunnel: w329 -> [_ w335]
              tunnel: w318 -> [_ w341]
              tunnel: w317 -> [_ w336]
              frame False {
              }
              frame True {
                n281 = call "Export Waveforms To Spreadsheet File with modified timestamps.vi"("file path (dialog if empty)"="MVC Filtered Path", "delimiter (Tab)"=", ", "waveforms"=w341, "trial start time"=w336, "append to file? (new file:F)"=TRUE, "header? (write header:T)"=FALSE) -> ()  [unwired: 8 in, 2 out]
                n282 = call "Export Waveforms To Spreadsheet File with modified timestamps.vi"("file path (dialog if empty)"="MVC Raw Path", "delimiter (Tab)"=", ", "waveforms"=w335, "trial start time"=w336, "append to file? (new file:F)"=TRUE, "header? (write header:T)"=FALSE) -> ()  [unwired: 8 in, 2 out]
              }
            }
            n283 = Index Array(array=w318, index=w328) -> (element=→"Current MVC (Filtered)":waveform(dbl))
            n284 = local read "MVC Duration (s)"() -> (w331:dbl)
            n285 = Get Date/Time In Seconds() -> (seconds since 1Jan1904=w326:timestamp)
            "mvc last time" <- w326
            n286 = Subtract(x=w326, y=w317) -> (x-y=w332:dbl)
            n287 = Greater Or Equal?(x=w332, y=w331) -> (x >= y?=w319:bool)
            n288 = case shown="True" w319 {
              frame False {
              }
              frame True {
                w345 = T2."Enabled" ("Disabled")
                n289 = local read "Collecting Data"() -> (w344:bool)
                n290 = local write "State"(T1."No Save" ("State")) -> ()
                n291 = property on="StartTrial" class="Bool (strict)"("DisabledEnum"=w345) -> ()  [unwired: 2 in, 2 out]
                n292 = property on="Set Parameters" class="Bool (strict)"("DisabledEnum"=w345) -> ()  [unwired: 2 in, 2 out]
                n293 = case shown="True" w344 {
                  frame False {
                  }
                  frame True {
                    n294 = local read "MVC Number"() -> (w348:dbl)
                    n295 = Increment(x=w348) -> (x+1=w347:dbl)
                    n296 = local write "MVC Number"(w347) -> ()
                  }
                }
              }
            }
          }
        }
        "FilteredAndRectified" <- w250
        n297 = local write "MVC Data"(w256) -> ()
        n298 = local write "Disp Data"(w255) -> ()
        "raw data" <- w247
      }
      frame Error {
        # "Return true for any case which should stop the loop."
      }
    }
  }
  n299 = Release Queue(queue=w5, error in (no error)=w4) -> ()  [unwired: 1 in, 3 out]
  n300 = while {
    stop <- w365 stop-if-true
    # "Update Display and Save Display Data"
    n301 = local read "loopTime"() -> (w364:dbl)
    n302 = local read "stop"() -> (w365:bool)
    n303 = local read "Disp Data"() -> (w368:cluster{"queue out":refnum<queue>, dbl, dbl}[])
    n304 = local read "enableSave"() -> (w355:bool)
    n305 = Wait (ms)(milliseconds to wait=w364) -> ()  [unwired: 1 out]
    n306 = local read "State"() -> (w356:T1)
    n307 = Index Array(array=w368, index="EMG Channel To Display") -> (element=w366:cluster{"queue out":refnum<queue>, dbl, dbl})
    n308 = Not Equal?(x=w356, y=T1."No Save" ("State")) -> (x != y?=w359:bool)
    n309 = Equal?(x=T1."Trial In Progress" ("State"), y=w356) -> (x = y?=w354:bool)
    n310 = Unbundle(w366) -> ("queue out"=w351:refnum<queue>, w352:dbl)  [unwired: 1 out]
    "DisplayBarActivation" <- w352
    "Current Activation" <- w352
    "Display Values" <- w352
    n311 = And(x=w354, y=w355) -> (x .and. y?=w353:bool)
    n312 = And(x=w359, y=w355) -> (x .and. y?=→"Collecting Data":bool)
    n313 = call "BarDisplay2Var.vi"("barOrGraph"="barOrGraph", "Activation Percentage"=w352, "scale min"="Display Min", "scale max"="Display Max", "Target Percentage"="Target Percentage") -> ()  [unwired: 7 in]
    n314 = case shown="True" w353 {
      tunnel: w352 -> [_ w375]
      frame False {
      }
      frame True {
        n315 = local read "RecordStartTime"() -> (w374:timestamp)
        n316 = Get Date/Time In Seconds() -> (seconds since 1Jan1904=w373:timestamp)
        n317 = Format Into String(w375) -> (resulting string=w371:string)  [unwired: 3 in, 1 out]
        n318 = Subtract(x=w373, y=w374) -> (x-y=w372:dbl)
        n319 = Format Into String(w372) -> (resulting string=w370:string)  [unwired: 3 in, 1 out]
        n320 = Build Array(w370, w371) -> (w377:string[])
        n321 = Build Array(w377) -> (w378:string[][])
        n322 = call-poly <vilib>:"Write Delimited Spreadsheet.vi"("file path (dialog if empty)"="trial display data", "2D data"=w378, "append to file? (new file:F)"=TRUE, "delimiter (\\t)"=", " ("delimiter (\\t)")) -> ()  [unwired: 10 in, 2 out]
      }
    }
    n323 = Get Queue Status(queue=w351) -> (# elements in queue=→"DispQueueSize":i32)  [unwired: 2 in, 7 out]
  }
